vi "Read Param control refs.vi"(8 "error in (no error)":errorcluster, 11 "UI in":refnum<class "CV-UI.lvclass">) -> (0 "error out":errorcluster, 2 "Param control refs":refnum<class "Param refs.lvclass">, 3 "UI out":refnum<class "CV-UI.lvclass">)   [LabVIEW 2013]
uses:
  CV-UI.lvclass
  Parameter control references/Param refs.lvclass
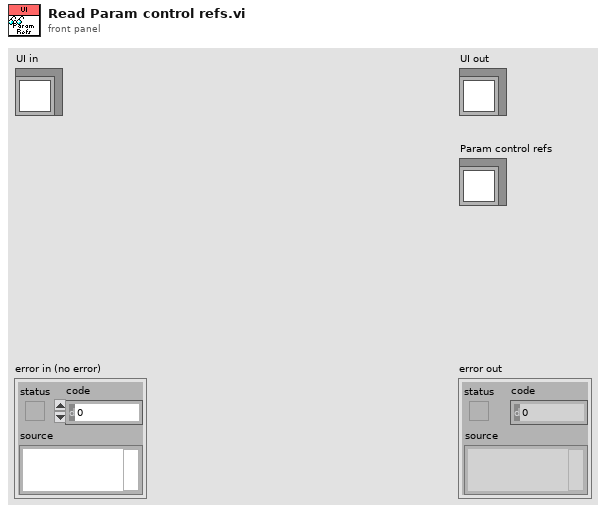
[diagram p1: front panel]
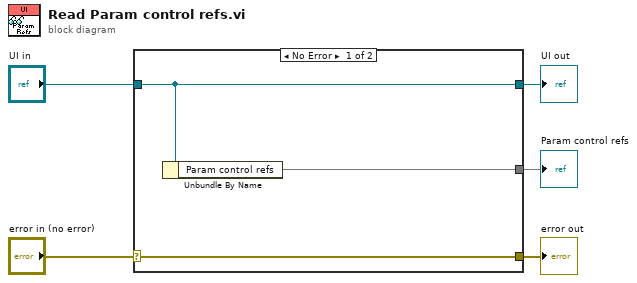
[diagram p0: block diagram]
diagram:
  n1 = case shown="No Error" "error in (no error)" {
    selector: "error in (no error)" -> [w8 w9]
    tunnel: [w8 w9] -> w4
    tunnel: [w7 w10] -> w2
    tunnel: "UI in" -> [w7 w10]
    tunnel: [w6 _] -> w1
    frame No Error {
      n2 = Unbundle By Name(w7) -> ("Param control refs"=w6)
    }
    frame Error {
    }
  }
  "error out" <- w4
  "UI out" <- w2
  "Param control refs" <- w1
